vi "preciovscostocafe.vi"(8 "error in (no error)":errorcluster, 11 "UI Actor in":refnum<class "UI Actor.lvclass">) -> (0 "error out":errorcluster, 3 "UI Actor out":refnum<class "UI Actor.lvclass">)   [LabVIEW 2019, in "UI Actor.lvlib" / "UI Actor.lvclass"]
uses:
  UI Actor.lvclass
  C:/Program Files (x86)/National Instruments/LabVIEW 2019/vi.lib/ActorFramework/Actor/Actor.lvclass
  UI Actor.lvclass/UI Actor.ctl
  Actor M Messages/Update M Msg/Update M Msg.lvclass/Update M Msg.ctl
  <vilib>/ActorFramework/Message Enqueuer/Message Enqueuer.lvclass/Message Enqueuer.ctl
  <vilib>/ActorFramework/Actor/Actor.lvclass/Actor.ctl
  UI Actor Messages/Credit update1 Msg/Credit update1 Msg.lvclass/Credit update1 Msg.ctl
  <vilib>/ActorFramework/Message Enqueuer/Enqueue.vi
  <vilib>/ActorFramework/Message Enqueuer/Init from Existing Queue.vi
  Actor M Messages/Update M Msg/Update M Msg.lvclass
  C:/Program Files (x86)/National Instruments/LabVIEW 2019/vi.lib/ActorFramework/Message/Message.lvclass
  UI Actor Messages/Credit update1 Msg/Credit update1 Msg.lvclass
  coffee Actor Messages/ActualizarTablacafe Msg/ActualizarTablacafe Msg.lvclass
  <vilib>/ActorFramework/Message Priority Queue/Priority Enqueue.vi
  <vilib>/ActorFramework/Message Enqueuer/Message Enqueuer.lvclass
  <vilib>/ActorFramework/Actor/Actor.lvclass
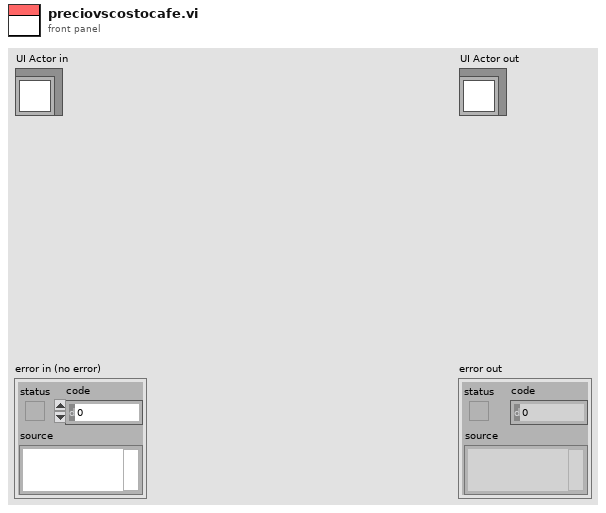
[diagram p1: front panel]
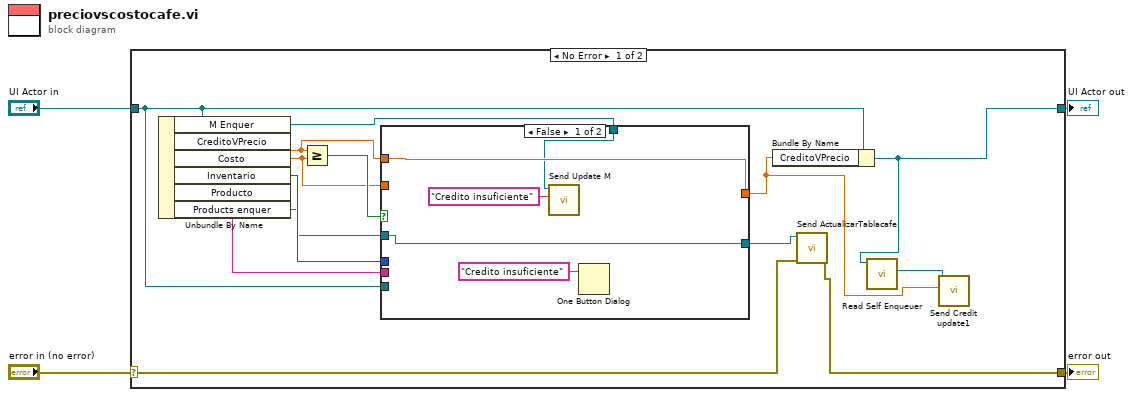
[diagram p0: block diagram]
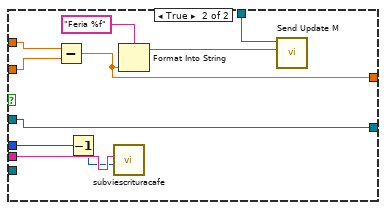
[diagram p2: hidden frame]
diagram:
  n1 = case shown="No Error" "error in (no error)" {
    selector: "error in (no error)" -> [w9 w35]
    tunnel: [w8 w35] -> w3
    tunnel: [w6 w34] -> w1
    tunnel: "UI Actor in" -> [w12 w34]
    frame No Error {
      n2 = Unbundle By Name(w12) -> ("M Enquer"=w13:refnum<class "Message Enqueuer.lvclass">, "CreditoVPrecio"=w16:dbl, "Costo"=w15:dbl, "Inventario"=w17:i32, "Producto"=w14:string, "Products enquer"=w11:refnum<class "Message Enqueuer.lvclass">)
      n3 = Greater Or Equal?(x=w16, y=w15) -> (x >= y?=w18:bool)
      n4 = case shown="False" w18 {
        tunnel: w17 -> [_ w33]
        tunnel: w16 -> [w23 w32]
        tunnel: w15 -> [_ w31]
        tunnel: w12 -> [_ _]
        tunnel: w14 -> [_ w25]
        tunnel: w13 -> [w20 w28]
        tunnel: [w23 w27] -> w5
        tunnel: w11 -> [w22 w26]
        tunnel: [w22 w26] -> w10
        frame False {
          n5 = call "Send Update M.vi"("Update M"="Credito insuficiente", "Message Enqueuer"=w20) -> ()  [unwired: 8 in, 2 out]
          n6 = One Button Dialog(message="Credito insuficiente") -> ()  [unwired: 1 in, 1 out]
        }
        frame True {
          n7 = Subtract(x=w32, y=w31) -> (x-y=w27:dbl)
          n8 = Decrement(x=w33) -> (x-1=w24:i32)
          n9 = call "subviescrituracafe.vi"("Numeric"=w24, "section"=w25) -> ()  [unwired: 10 in]
          n10 = Format Into String "Format Into String"(format string="Feria %f", w27) -> (resulting string=w29:string)  [unwired: 2 in, 1 out]
          n11 = call "Send Update M.vi"("Update M"=w29, "Message Enqueuer"=w28) -> ()  [unwired: 8 in, 2 out]
        }
      }
      n12 = Bundle By Name(cluster=w12, "CreditoVPrecio"=w5) -> (w6:refnum<class "UI Actor.lvclass">)
      n13 = call "Send ActualizarTablacafe.vi"("error in (no error)"=w9, "Message Enqueuer"=w10) -> ("error out"=w8:errorcluster)  [unwired: 8 in, 1 out]
      n14 = call <vilib>:"Read Self Enqueuer.vi"("Actor"=w6) -> ("Self Enqueuer"=w7:refnum<class "Message Enqueuer.lvclass">)  [unwired: 10 in]
      n15 = call "Send Credit update1.vi"("Credit"=w5, "Message Enqueuer"=w7) -> ()  [unwired: 8 in, 2 out]
    }
    frame Error {
    }
  }
  "error out" <- w3
  "UI Actor out" <- w1
